vi "CAN总线测试.vi"() -> ()   [LabVIEW 2010]
panel:
  in  "同步_2":i32
  in  "同步_1":i32
  out "CAN_R_4_4":u16
  out "CAN_R_4_3":u16
  out "CAN_R_4_2":u16
  out "CAN_R_4_1":u16
  out "CAN_R_3_4":u16
  out "CAN_R_3_3":u16
  out "CAN_R_3_2":u16
  out "CAN_R_3_1":u16
  out "CAN_R_2_4":u16
  out "CAN_R_2_3":u16
  out "CAN_R_2_2":u16
  out "CAN_R_2_1":u16
  out "CAN_R_1_4":u16
  out "CAN_R_1_3":u16
  out "CAN_R_1_2":u16
  out "CAN_R_1_1":u16
  out "结束?":bool
  out "light_4":bool
  out "light_3":bool
  out "light_2":bool
  out "light_1":bool
  out "测试结论":string
  in  "btn_关闭":bool
  in  "btn_开始测试":bool
  in  "CAN_4_4":u16
  in  "CAN_4_3":u16
  in  "CAN_4_2":u16
  in  "CAN_4_1":u16
  in  "单选_CAN_4":bool
  in  "CAN_3_4":u16
  in  "CAN_3_3":u16
  in  "CAN_3_2":u16
  in  "CAN_3_1":u16
  in  "单选_CAN_3":bool
  in  "CAN_2_4":u16
  in  "CAN_2_3":u16
  in  "CAN_2_2":u16
  in  "CAN_2_1":u16
  in  "单选_CAN_2":bool
  in  "CAN_1_4":u16
  in  "CAN_1_3":u16
  in  "CAN_1_2":u16
  in  "CAN_1_1":u16
  in  "单选_CAN_1":bool
  # "CAN以发送数据："
  # "CAN1"
  # "CAN2"
  # "CAN3"
  # "CAN4"
  # "CAN接收数据："
  # "CAN1"
  # "CAN2"
  # "CAN3"
  # "CAN4"
  # "测试结论："
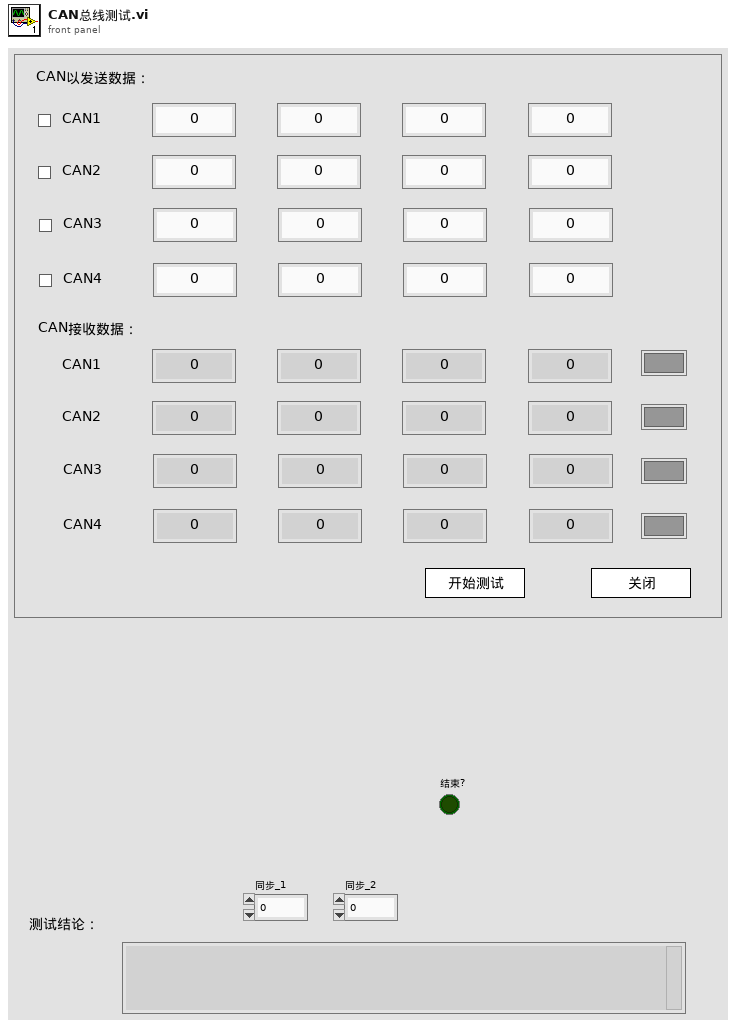
[diagram p1: front panel]
types:
  T1 = enum8{"Enabled", "Disabled", "Disabled and Grayed Out"}
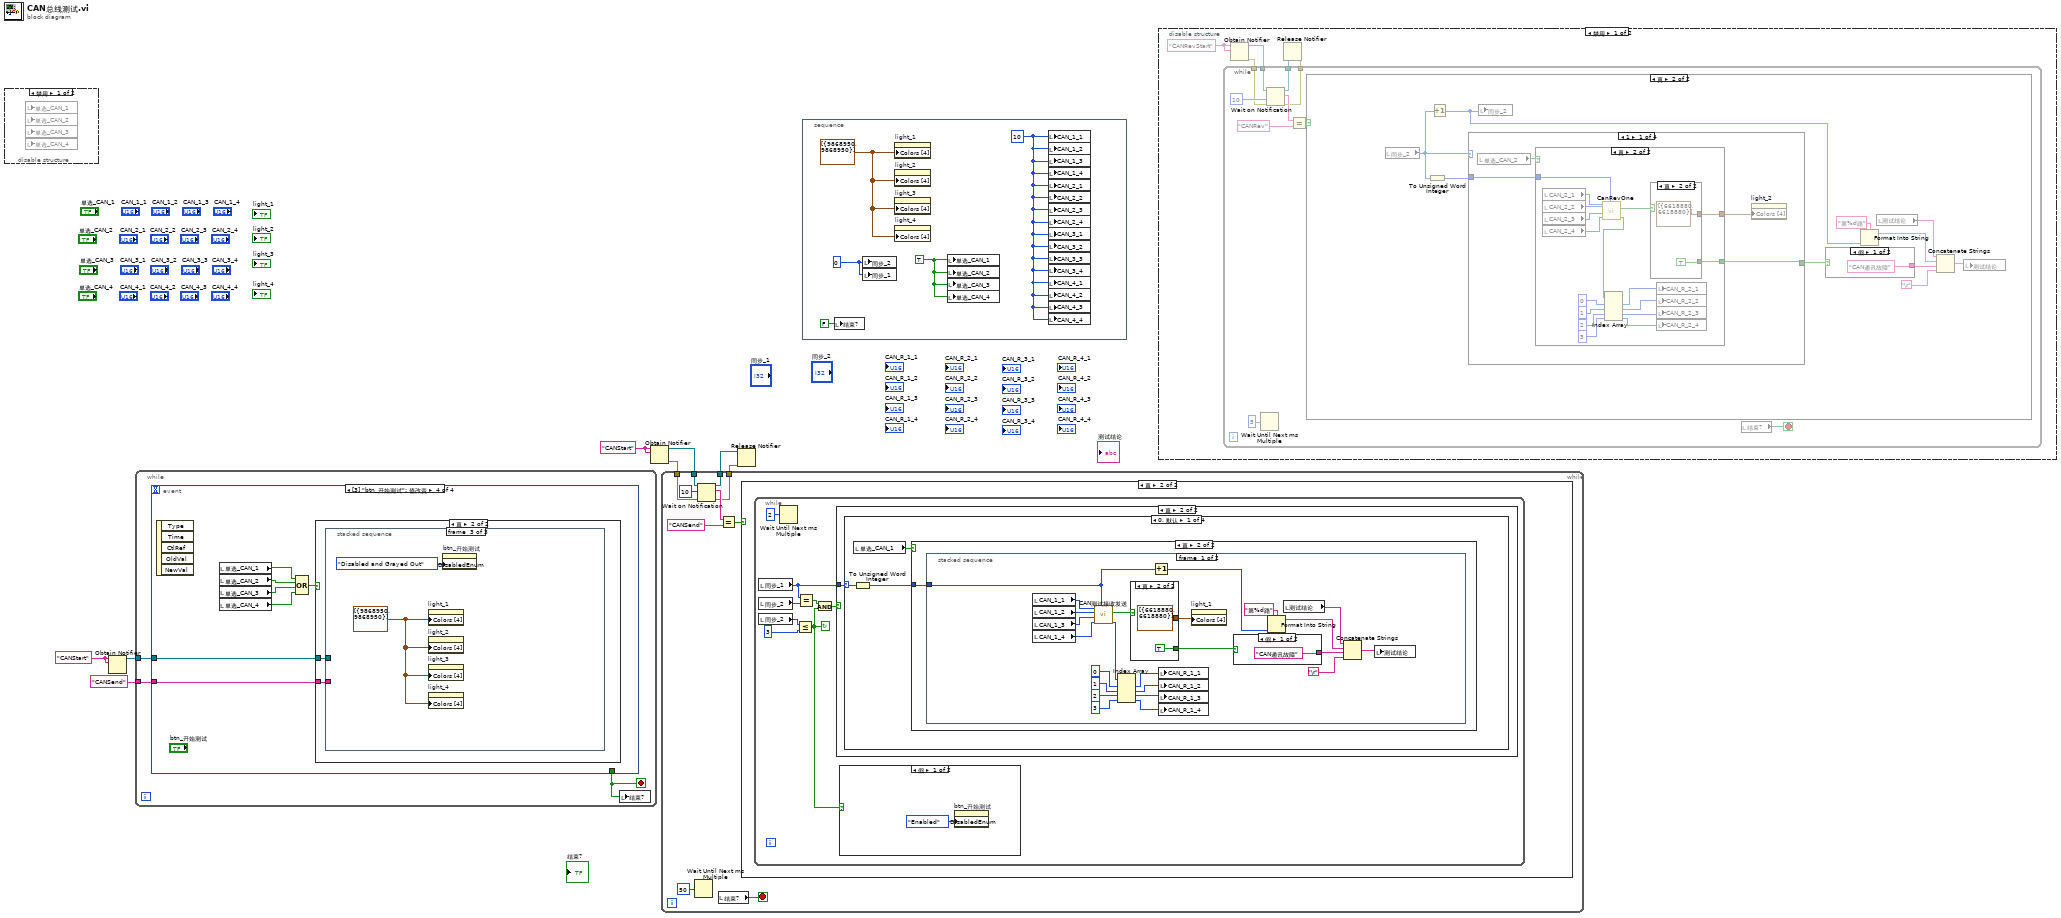
[diagram p0: block diagram]
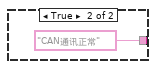
[diagram p3: hidden frame]
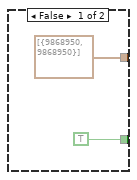
[diagram p4: hidden frame]
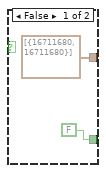
[diagram p5: hidden frame]
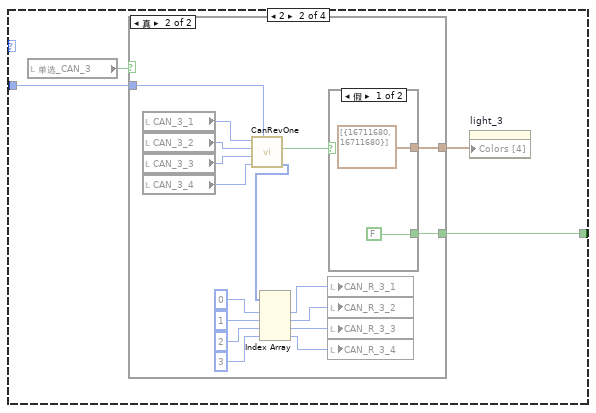
[diagram p6: hidden frame]
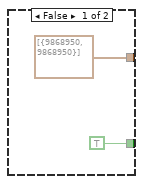
[diagram p7: hidden frame]
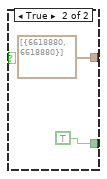
[diagram p8: hidden frame]
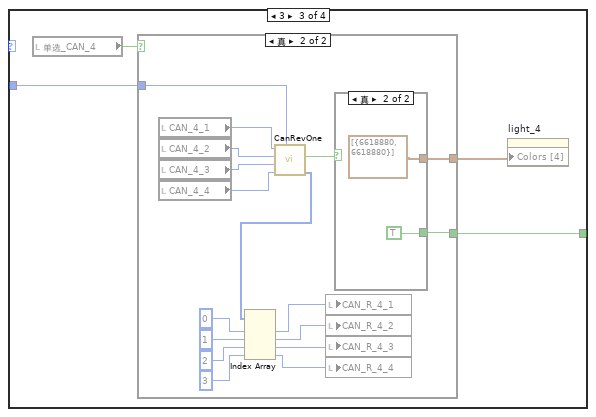
[diagram p9: hidden frame]
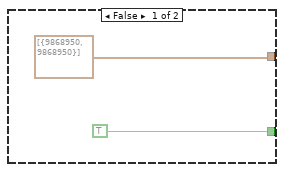
[diagram p10: hidden frame]
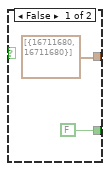
[diagram p11: hidden frame]
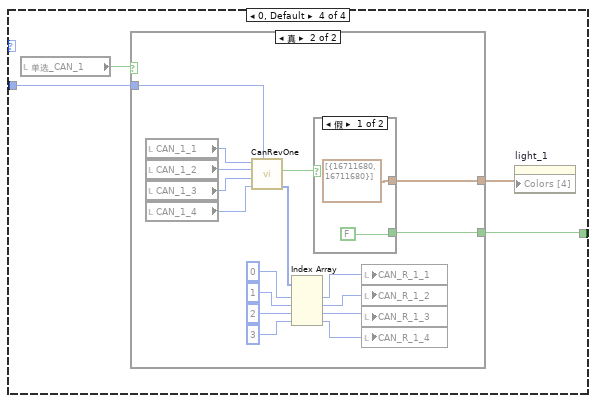
[diagram p12: hidden frame]
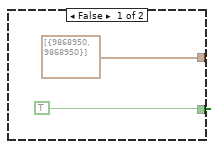
[diagram p13: hidden frame]
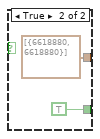
[diagram p14: hidden frame]
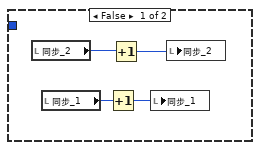
[diagram p19: hidden frame]
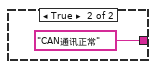
[diagram p20: hidden frame]
diagram:
  w3 = "CANStart" ("名称（未命名）")
  w8 = "CANStart" ("名称（未命名）")
  n1 = disable-structure shown="禁用" {
    frame Disabled {
      n2 = local read "单选_CAN_1"() -> ()  [unwired: 1 in]
      n3 = local read "单选_CAN_2"() -> ()  [unwired: 1 in]
      n4 = local read "单选_CAN_3"() -> ()  [unwired: 1 in]
      n5 = local read "单选_CAN_4"() -> ()  [unwired: 1 in]
    }
    frame Enabled {
    }
  }
  n6 = Obtain Notifier(name (unnamed)=w3, notification data type=w3) -> (notifier out=w2:refnum<notifier>)  [unwired: 2 in, 2 out]
  n7 = while {
    tunnel: w2 -> [w10]
    tunnel: "CANSend" ("通知") -> [w9]
    stop <- w11 stop-if-true
    n8 = event shown="[3] \"btn_开始测试\": 值改变" {
      selector: _ -> [_ _ _ _]
      dyn-events: _ -> [_ _ _ _]
      timeout: _ -> [_ _ _ _]
      tunnel: [_ TRUE TRUE _] -> w11
      tunnel: w10 -> [_ _ _ w21]
      tunnel: w9 -> [_ _ _ w20]
      event Timeout {
        n9 = event-data() -> ()  [unwired: 1 in, 2 out]
      }
      event Panel Close {
        n10 = event-data() -> ()  [unwired: 1 in, 3 out]
        n11 = stacked-sequence {
          frame #0 {
            w13 = u16 0 ("CAN_R_1_1")
            w14 = 0 ("同步_2")
            w15 = cluster{u32, u32}[] [{9868950, 9868950}]
            n12 = local write "同步_2"(w14) -> ()
            n13 = local write "同步_1"(w14) -> ()
            n14 = property on="light_1" class="Bool (严格)"("Colors [4]"=w15) -> ()  [unwired: 2 in, 2 out]
            n15 = property on="light_2" class="Bool (严格)"("Colors [4]"=w15) -> ()  [unwired: 2 in, 2 out]
            n16 = property on="light_3" class="Bool (严格)"("Colors [4]"=w15) -> ()  [unwired: 2 in, 2 out]
            n17 = property on="light_4" class="Bool (严格)"("Colors [4]"=w15) -> ()  [unwired: 2 in, 2 out]
            n18 = local write "CAN_R_1_1"(w13) -> ()
            n19 = local write "CAN_R_1_2"(w13) -> ()
            n20 = local write "CAN_R_1_3"(w13) -> ()
            n21 = local write "CAN_R_1_4"(w13) -> ()
            n22 = local write "CAN_R_2_1"(w13) -> ()
            n23 = local write "CAN_R_2_2"(w13) -> ()
            n24 = local write "CAN_R_2_3"(w13) -> ()
            n25 = local write "CAN_R_2_4"(w13) -> ()
            n26 = local write "CAN_R_3_1"(w13) -> ()
            n27 = local write "CAN_R_3_2"(w13) -> ()
            n28 = local write "CAN_R_3_3"(w13) -> ()
            n29 = local write "CAN_R_3_4"(w13) -> ()
            n30 = local write "CAN_R_4_1"(w13) -> ()
            n31 = local write "CAN_R_4_2"(w13) -> ()
            n32 = local write "CAN_R_4_3"(w13) -> ()
            n33 = local write "CAN_R_4_4"(w13) -> ()
          }
        }
      }
      event "btn_关闭": Value Change {
        n34 = event-data() -> ()  [unwired: 1 in, 5 out]
        n35 = stacked-sequence {
          frame #0 {
            w17 = u16 0 ("CAN_R_1_1")
            w18 = 0 ("同步_2")
            w19 = cluster{u32, u32}[] [{9868950, 9868950}]
            n36 = local write "同步_2"(w18) -> ()
            n37 = local write "同步_1"(w18) -> ()
            n38 = property on="light_1" class="Bool (严格)"("Colors [4]"=w19) -> ()  [unwired: 2 in, 2 out]
            n39 = property on="light_2" class="Bool (严格)"("Colors [4]"=w19) -> ()  [unwired: 2 in, 2 out]
            n40 = property on="light_3" class="Bool (严格)"("Colors [4]"=w19) -> ()  [unwired: 2 in, 2 out]
            n41 = property on="light_4" class="Bool (严格)"("Colors [4]"=w19) -> ()  [unwired: 2 in, 2 out]
            n42 = local write "CAN_R_1_1"(w17) -> ()
            n43 = local write "CAN_R_1_2"(w17) -> ()
            n44 = local write "CAN_R_1_3"(w17) -> ()
            n45 = local write "CAN_R_1_4"(w17) -> ()
            n46 = local write "CAN_R_2_1"(w17) -> ()
            n47 = local write "CAN_R_2_2"(w17) -> ()
            n48 = local write "CAN_R_2_3"(w17) -> ()
            n49 = local write "CAN_R_2_4"(w17) -> ()
            n50 = local write "CAN_R_3_1"(w17) -> ()
            n51 = local write "CAN_R_3_2"(w17) -> ()
            n52 = local write "CAN_R_3_3"(w17) -> ()
            n53 = local write "CAN_R_3_4"(w17) -> ()
            n54 = local write "CAN_R_4_1"(w17) -> ()
            n55 = local write "CAN_R_4_2"(w17) -> ()
            n56 = local write "CAN_R_4_3"(w17) -> ()
            n57 = local write "CAN_R_4_4"(w17) -> ()
          }
        }
      }
      event "btn_开始测试": Value Change {
        n58 = event-data() -> ()  [unwired: 1 in, 5 out]
        n59 = local read "单选_CAN_1"() -> (w26:bool)
        n60 = local read "单选_CAN_2"() -> (w25:bool)
        n61 = local read "单选_CAN_3"() -> (w24:bool)
        n62 = local read "单选_CAN_4"() -> (w23:bool)
        n63 = Compound Arithmetic op=OR(w26, w25, w24, w23) -> (w22:bool)
        n64 = case shown="真" w22 {
          tunnel: w21 -> [_ w28]
          tunnel: w20 -> [_ w27]
          frame False {
            n65 = call "显示对话框信息"() -> ()  [unwired: 10 in, 2 out]
          }
          frame True {
            n66 = stacked-sequence {
              tunnel: w28 -> [_ w33 _]
              tunnel: w27 -> [_ w32 _]
              frame #0 {
                w29 = u16 0 ("CAN_R_1_1")
                w30 = 0 ("同步_2")
                n67 = local write "同步_2"(w30) -> ()
                n68 = local write "同步_1"(w30) -> ()
                n69 = local write "测试结论"("") -> ()
                n70 = local write "CAN_R_1_1"(w29) -> ()
                n71 = local write "CAN_R_1_2"(w29) -> ()
                n72 = local write "CAN_R_1_3"(w29) -> ()
                n73 = local write "CAN_R_1_4"(w29) -> ()
                n74 = local write "CAN_R_2_1"(w29) -> ()
                n75 = local write "CAN_R_2_2"(w29) -> ()
                n76 = local write "CAN_R_2_3"(w29) -> ()
                n77 = local write "CAN_R_2_4"(w29) -> ()
                n78 = local write "CAN_R_3_1"(w29) -> ()
                n79 = local write "CAN_R_3_2"(w29) -> ()
                n80 = local write "CAN_R_3_3"(w29) -> ()
                n81 = local write "CAN_R_3_4"(w29) -> ()
                n82 = local write "CAN_R_4_1"(w29) -> ()
                n83 = local write "CAN_R_4_2"(w29) -> ()
                n84 = local write "CAN_R_4_3"(w29) -> ()
                n85 = local write "CAN_R_4_4"(w29) -> ()
              }
              frame #1 {
                n86 = Send Notification(notification=w32, notifier=w33) -> ()  [unwired: 1 in, 2 out]
              }
              frame #2 {
                w34 = cluster{u32, u32}[] [{9868950, 9868950}]
                n87 = property on="light_1" class="Bool (严格)"("Colors [4]"=w34) -> ()  [unwired: 2 in, 2 out]
                n88 = property on="light_2" class="Bool (严格)"("Colors [4]"=w34) -> ()  [unwired: 2 in, 2 out]
                n89 = property on="light_3" class="Bool (严格)"("Colors [4]"=w34) -> ()  [unwired: 2 in, 2 out]
                n90 = property on="light_4" class="Bool (严格)"("Colors [4]"=w34) -> ()  [unwired: 2 in, 2 out]
                n91 = property on="btn_开始测试" class="Bool"("DisabledEnum"=T1."Disabled and Grayed Out" ("禁用")) -> ()  [unwired: 2 in, 2 out]
              }
            }
          }
        }
      }
    }
    n92 = local write "结束?"(w11) -> ()
  }
  n93 = Obtain Notifier(name (unnamed)=w8, notification data type=w8) -> (notifier out=w6:refnum<notifier>, error out=w7:errorcluster)  [unwired: 2 in, 1 out]
  n94 = while {
    tunnel: w7 -> [w39]
    tunnel: w6 -> [w38]
    tunnel: [w37] -> w5
    tunnel: [w36] -> w4
    stop <- w44 stop-if-true
    n95 = Wait Until Next ms Multiple(millisecond multiple=u32 50 ("毫秒倍数")) -> ()  [unwired: 1 out]
    n96 = Wait on Notification(notifier=w38, timeout in ms (-1)=10 ("超时毫秒(-1)"), error in (no error)=w39) -> (notifier out=w37:refnum<notifier>, notification=w41:string, error out=w36:errorcluster)  [unwired: 1 in, 1 out]
    n97 = local read "结束?"() -> (w44:bool)
    n98 = Equal?(x=w41, y="CANSend" ("通知")) -> (x = y?=w40:bool)
    n99 = case shown="真" w40 {
      frame False {
      }
      frame True {
        n100 = while {
          stop <- w46 continue-if-true
          n101 = local read "同步_1"() -> (w53:i32)
          n102 = local read "同步_2"() -> (w49:i32)
          n103 = local read "同步_2"() -> (w51:i32)
          n104 = Wait Until Next ms Multiple(millisecond multiple=u32 2 ("毫秒倍数")) -> ()  [unwired: 1 out]
          n105 = Less Or Equal?(x=w51, y=3) -> (x <= y?=w46:bool)
          n106 = Equal?(x=w53, y=w49) -> (x = y?=w47:bool)
          n107 = And(x=w47, y=w46) -> (x .and. y?=w48:bool)
          n108 = case shown="真" w48 {
            tunnel: w53 -> [_ w55]
            frame False {
            }
            frame True {
              n109 = case shown="0, 默认" w55 {
                selector: w55 -> [w56 w100 w142 w184]
                frame 0, Default {
                  n110 = local read "单选_CAN_1"() -> (w58:bool)
                  n111 = To Unsigned Word Integer(number=w56) -> (unsigned 16bit integer=w57:u16)
                  n112 = case shown="真" w58 {
                    tunnel: w57 -> [_ w63]
                    frame False {
                      n113 = local read "同步_2"() -> (w61:i32)
                      n114 = local read "同步_1"() -> (w59:i32)
                      n115 = Increment(x=w59) -> (x+1=w60:i32)
                      n116 = Increment(x=w61) -> (x+1=w62:i32)
                      n117 = local write "同步_1"(w60) -> ()
                      n118 = local write "同步_2"(w62) -> ()
                    }
                    frame True {
                      n119 = stacked-sequence {
                        tunnel: w63 -> [w64 _]
                        frame #0 {
                          n120 = local read "CAN_1_1"() -> (w74:u16)
                          n121 = local read "CAN_1_2"() -> (w75:u16)
                          n122 = local read "CAN_1_3"() -> (w76:u16)
                          n123 = local read "CAN_1_4"() -> (w77:u16)
                          n124 = call "CAN测试接收发送.vi"("Order"=w64, "data_4"=w77, "data_3"=w76, "data_2"=w75, "data_1"=w74) -> ("接收数据"=w79:u16[], "成功？"=w78:bool)  [unwired: 5 in]
                          n125 = Index Array(array=w79, index #1=0 ("索引"), index #2=1 ("索引"), index #3=2 ("索引"), index #4=3 ("索引")) -> (element #1=w84:u16, element #2=w85:u16, element #3=w86:u16, element #4=w87:u16)
                          n126 = case shown="真" w78 {
                            tunnel: [cluster{u32, u32}[] [{16711680, 16711680}] cluster{u32, u32}[] [{6618880, 6618880}]] -> w73
                            tunnel: [FALSE TRUE] -> w65
                            frame False {
                            }
                            frame True {
                            }
                          }
                          n127 = Increment(x=w64) -> (x+1=w66:u16)
                          n128 = local write "CAN_R_1_1"(w84) -> ()
                          n129 = local write "CAN_R_1_2"(w85) -> ()
                          n130 = local write "CAN_R_1_3"(w86) -> ()
                          n131 = local write "CAN_R_1_4"(w87) -> ()
                          n132 = property on="light_1" class="Bool (严格)"("Colors [4]"=w73) -> ()  [unwired: 2 in, 2 out]
                          n133 = case shown="假" w65 {
                            tunnel: ["CAN通讯故障" "CAN通讯正常"] -> w69
                            frame False {
                            }
                            frame True {
                            }
                          }
                          n134 = Format Into String(format string="第%d路", w66) -> (resulting string=w70:string)  [unwired: 2 in, 1 out]
                          n135 = local read "测试结论"() -> (w71:string)
                          n136 = Concatenate Strings(w71, w70, w69, "\r") -> (w67:string)
                          n137 = local write "测试结论"(w67) -> ()
                        }
                        frame #1 {
                          n138 = local read "同步_1"() -> (w96:i32)
                          n139 = local read "同步_2"() -> (w94:i32)
                          n140 = Increment(x=w96) -> (x+1=w97:i32)
                          n141 = Increment(x=w94) -> (x+1=w95:i32)
                          n142 = local write "同步_2"(w95) -> ()
                          n143 = local write "同步_1"(w97) -> ()
                        }
                      }
                    }
                  }
                }
                frame 1 {
                  n144 = local read "单选_CAN_2"() -> (w99:bool)
                  n145 = To Unsigned Word Integer(number=w100) -> (unsigned 16bit integer=w98:u16)
                  n146 = case shown="真" w99 {
                    tunnel: w98 -> [_ w105]
                    frame False {
                      n147 = local read "同步_2"() -> (w103:i32)
                      n148 = local read "同步_1"() -> (w101:i32)
                      n149 = Increment(x=w101) -> (x+1=w102:i32)
                      n150 = Increment(x=w103) -> (x+1=w104:i32)
                      n151 = local write "同步_1"(w102) -> ()
                      n152 = local write "同步_2"(w104) -> ()
                    }
                    frame True {
                      n153 = stacked-sequence {
                        tunnel: w105 -> [w129 _]
                        frame #0 {
                          n154 = local read "CAN_2_1"() -> (w115:u16)
                          n155 = local read "CAN_2_2"() -> (w116:u16)
                          n156 = local read "CAN_2_3"() -> (w117:u16)
                          n157 = local read "CAN_2_4"() -> (w118:u16)
                          n158 = call "CAN测试接收发送.vi"("Order"=w129, "data_4"=w118, "data_3"=w117, "data_2"=w116, "data_1"=w115) -> ("接收数据"=w124:u16[], "成功？"=w119:bool)  [unwired: 5 in]
                          n159 = Index Array(array=w124, index #1=0 ("索引"), index #2=1 ("索引"), index #3=2 ("索引"), index #4=3 ("索引")) -> (element #1=w125:u16, element #2=w126:u16, element #3=w127:u16, element #4=w128:u16)
                          n160 = case shown="真" w119 {
                            tunnel: [cluster{u32, u32}[] [{16711680, 16711680}] cluster{u32, u32}[] [{6618880, 6618880}]] -> w114
                            tunnel: [FALSE TRUE] -> w107
                            frame False {
                            }
                            frame True {
                            }
                          }
                          n161 = local write "CAN_R_2_1"(w125) -> ()
                          n162 = local write "CAN_R_2_2"(w126) -> ()
                          n163 = local write "CAN_R_2_3"(w127) -> ()
                          n164 = local write "CAN_R_2_4"(w128) -> ()
                          n165 = Increment(x=w129) -> (x+1=w106:u16)
                          n166 = property on="light_2" class="Bool (严格)"("Colors [4]"=w114) -> ()  [unwired: 2 in, 2 out]
                          n167 = case shown="假" w107 {
                            tunnel: ["CAN通讯故障" "CAN通讯正常"] -> w111
                            frame False {
                            }
                            frame True {
                            }
                          }
                          n168 = Format Into String(format string="第%d路", w106) -> (resulting string=w110:string)  [unwired: 2 in, 1 out]
                          n169 = local read "测试结论"() -> (w109:string)
                          n170 = Concatenate Strings(w109, w110, w111, "\r") -> (w113:string)
                          n171 = local write "测试结论"(w113) -> ()
                        }
                        frame #1 {
                          n172 = local read "同步_1"() -> (w138:i32)
                          n173 = local read "同步_2"() -> (w137:i32)
                          n174 = Increment(x=w138) -> (x+1=w139:i32)
                          n175 = Increment(x=w137) -> (x+1=w136:i32)
                          n176 = local write "同步_2"(w136) -> ()
                          n177 = local write "同步_1"(w139) -> ()
                        }
                      }
                    }
                  }
                }
                frame 2 {
                  n178 = local read "单选_CAN_3"() -> (w141:bool)
                  n179 = To Unsigned Word Integer(number=w142) -> (unsigned 16bit integer=w140:u16)
                  n180 = case shown="真" w141 {
                    tunnel: w140 -> [_ w147]
                    frame False {
                      n181 = local read "同步_1"() -> (w143:i32)
                      n182 = local read "同步_2"() -> (w145:i32)
                      n183 = Increment(x=w143) -> (x+1=w144:i32)
                      n184 = Increment(x=w145) -> (x+1=w146:i32)
                      n185 = local write "同步_1"(w144) -> ()
                      n186 = local write "同步_2"(w146) -> ()
                    }
                    frame True {
                      n187 = stacked-sequence {
                        tunnel: w147 -> [w171 _]
                        frame #0 {
                          n188 = local read "CAN_3_1"() -> (w157:u16)
                          n189 = local read "CAN_3_2"() -> (w158:u16)
                          n190 = local read "CAN_3_3"() -> (w159:u16)
                          n191 = local read "CAN_3_4"() -> (w160:u16)
                          n192 = call "CAN测试接收发送.vi"("Order"=w171, "data_4"=w160, "data_3"=w159, "data_2"=w158, "data_1"=w157) -> ("接收数据"=w166:u16[], "成功？"=w161:bool)  [unwired: 5 in]
                          n193 = Index Array(array=w166, index #1=0 ("索引"), index #2=1 ("索引"), index #3=2 ("索引"), index #4=3 ("索引")) -> (element #1=w167:u16, element #2=w168:u16, element #3=w169:u16, element #4=w170:u16)
                          n194 = local write "CAN_R_3_1"(w167) -> ()
                          n195 = local write "CAN_R_3_2"(w168) -> ()
                          n196 = local write "CAN_R_3_3"(w169) -> ()
                          n197 = local write "CAN_R_3_4"(w170) -> ()
                          n198 = case shown="真" w161 {
                            tunnel: [cluster{u32, u32}[] [{16711680, 16711680}] cluster{u32, u32}[] [{6618880, 6618880}]] -> w156
                            tunnel: [FALSE TRUE] -> w148
                            frame False {
                            }
                            frame True {
                            }
                          }
                          n199 = Increment(x=w171) -> (x+1=w149:u16)
                          n200 = property on="light_3" class="Bool (严格)"("Colors [4]"=w156) -> ()  [unwired: 2 in, 2 out]
                          n201 = case shown="假" w148 {
                            tunnel: ["CAN通讯故障" "CAN通讯正常"] -> w153
                            frame False {
                            }
                            frame True {
                            }
                          }
                          n202 = Format Into String(format string="第%d路", w149) -> (resulting string=w152:string)  [unwired: 2 in, 1 out]
                          n203 = local read "测试结论"() -> (w151:string)
                          n204 = Concatenate Strings(w151, w152, w153, "\r") -> (w155:string)
                          n205 = local write "测试结论"(w155) -> ()
                        }
                        frame #1 {
                          n206 = local read "同步_1"() -> (w180:i32)
                          n207 = local read "同步_2"() -> (w178:i32)
                          n208 = Increment(x=w180) -> (x+1=w181:i32)
                          n209 = Increment(x=w178) -> (x+1=w179:i32)
                          n210 = local write "同步_1"(w181) -> ()
                          n211 = local write "同步_2"(w179) -> ()
                        }
                      }
                    }
                  }
                }
                frame 3 {
                  n212 = local read "单选_CAN_4"() -> (w183:bool)
                  n213 = To Unsigned Word Integer(number=w184) -> (unsigned 16bit integer=w182:u16)
                  n214 = case shown="真" w183 {
                    tunnel: w182 -> [_ w189]
                    frame False {
                      n215 = local read "同步_2"() -> (w187:i32)
                      n216 = local read "同步_1"() -> (w186:i32)
                      n217 = Increment(x=w187) -> (x+1=w188:i32)
                      n218 = Increment(x=w186) -> (x+1=w185:i32)
                      n219 = local write "同步_1"(w185) -> ()
                      n220 = local write "同步_2"(w188) -> ()
                    }
                    frame True {
                      n221 = stacked-sequence {
                        tunnel: w189 -> [w213 _]
                        frame #0 {
                          n222 = local read "CAN_4_1"() -> (w212:u16)
                          n223 = local read "CAN_4_2"() -> (w211:u16)
                          n224 = local read "CAN_4_3"() -> (w210:u16)
                          n225 = local read "CAN_4_4"() -> (w209:u16)
                          n226 = call "CAN测试接收发送.vi"("Order"=w213, "data_4"=w209, "data_3"=w210, "data_2"=w211, "data_1"=w212) -> ("接收数据"=w203:u16[], "成功？"=w208:bool)  [unwired: 5 in]
                          n227 = Index Array(array=w203, index #1=0 ("索引"), index #2=1 ("索引"), index #3=2 ("索引"), index #4=3 ("索引")) -> (element #1=w202:u16, element #2=w201:u16, element #3=w200:u16, element #4=w199:u16)
                          n228 = local write "CAN_R_4_1"(w202) -> ()
                          n229 = local write "CAN_R_4_2"(w201) -> ()
                          n230 = local write "CAN_R_4_3"(w200) -> ()
                          n231 = local write "CAN_R_4_4"(w199) -> ()
                          n232 = case shown="真" w208 {
                            tunnel: [cluster{u32, u32}[] [{16711680, 16711680}] cluster{u32, u32}[] [{6618880, 6618880}]] -> w198
                            tunnel: [FALSE TRUE] -> w190
                            frame False {
                            }
                            frame True {
                            }
                          }
                          n233 = Increment(x=w213) -> (x+1=w191:u16)
                          n234 = property on="light_4" class="Bool (严格)"("Colors [4]"=w198) -> ()  [unwired: 2 in, 2 out]
                          n235 = case shown="假" w190 {
                            tunnel: ["CAN通讯故障" "CAN通讯正常"] -> w195
                            frame False {
                            }
                            frame True {
                            }
                          }
                          n236 = Format Into String(format string="第%d路", w191) -> (resulting string=w194:string)  [unwired: 2 in, 1 out]
                          n237 = local read "测试结论"() -> (w193:string)
                          n238 = Concatenate Strings(w193, w194, w195, "\r") -> (w197:string)
                          n239 = local write "测试结论"(w197) -> ()
                        }
                        frame #1 {
                          n240 = local read "同步_1"() -> (w223:i32)
                          n241 = local read "同步_2"() -> (w220:i32)
                          n242 = Increment(x=w223) -> (x+1=w222:i32)
                          n243 = Increment(x=w220) -> (x+1=w221:i32)
                          n244 = local write "同步_2"(w221) -> ()
                          n245 = local write "同步_1"(w222) -> ()
                        }
                      }
                    }
                  }
                }
              }
            }
          }
          n246 = case shown="假" w46 {
            frame False {
              n247 = property on="btn_开始测试" class="Bool"("DisabledEnum"=T1."Enabled" ("禁用")) -> ()  [unwired: 2 in, 2 out]
            }
            frame True {
            }
          }
        }
      }
    }
  }
  n248 = Release Notifier(notifier=w5, error in (no error)=w4) -> ()  [unwired: 1 in, 3 out]
  n249 = stacked-sequence {
    frame #0 {
      w224 = TRUE ("单选_CAN_1")
      w225 = u16 10 ("CAN_R_1_1")
      w226 = 0 ("同步_2")
      w228 = cluster{u32, u32}[] [{9868950, 9868950}]
      n250 = local write "结束?"(FALSE ("结束?")) -> ()
      n251 = local write "同步_2"(w226) -> ()
      n252 = local write "同步_1"(w226) -> ()
      n253 = property on="light_1" class="Bool (严格)"("Colors [4]"=w228) -> ()  [unwired: 2 in, 2 out]
      n254 = property on="light_2" class="Bool (严格)"("Colors [4]"=w228) -> ()  [unwired: 2 in, 2 out]
      n255 = property on="light_3" class="Bool (严格)"("Colors [4]"=w228) -> ()  [unwired: 2 in, 2 out]
      n256 = property on="light_4" class="Bool (严格)"("Colors [4]"=w228) -> ()  [unwired: 2 in, 2 out]
      n257 = local write "单选_CAN_1"(w224) -> ()
      n258 = local write "单选_CAN_2"(w224) -> ()
      n259 = local write "单选_CAN_3"(w224) -> ()
      n260 = local write "单选_CAN_4"(w224) -> ()
      n261 = local write "CAN_1_1"(w225) -> ()
      n262 = local write "CAN_1_2"(w225) -> ()
      n263 = local write "CAN_1_3"(w225) -> ()
      n264 = local write "CAN_1_4"(w225) -> ()
      n265 = local write "CAN_2_1"(w225) -> ()
      n266 = local write "CAN_2_2"(w225) -> ()
      n267 = local write "CAN_2_3"(w225) -> ()
      n268 = local write "CAN_2_4"(w225) -> ()
      n269 = local write "CAN_3_1"(w225) -> ()
      n270 = local write "CAN_3_2"(w225) -> ()
      n271 = local write "CAN_3_3"(w225) -> ()
      n272 = local write "CAN_3_4"(w225) -> ()
      n273 = local write "CAN_4_1"(w225) -> ()
      n274 = local write "CAN_4_2"(w225) -> ()
      n275 = local write "CAN_4_3"(w225) -> ()
      n276 = local write "CAN_4_4"(w225) -> ()
    }
  }
  n277 = disable-structure shown="禁用" {
    frame Disabled {
      w233 = "CANRevStart" ("名称（未命名）")
      n278 = Obtain Notifier(name (unnamed)=w233, notification data type=w233) -> (notifier out=w231:refnum<notifier>, error out=w232:errorcluster)  [unwired: 2 in, 1 out]
      n279 = while {
        tunnel: w232 -> [w238]
        tunnel: w231 -> [w237]
        tunnel: [w236] -> w230
        tunnel: [w235] -> w229
        stop <- w243 stop-if-true
        n280 = Wait Until Next ms Multiple(millisecond multiple=u32 5 ("毫秒倍数")) -> ()  [unwired: 1 out]
        n281 = Wait on Notification(notifier=w237, timeout in ms (-1)=10 ("超时毫秒(-1)"), error in (no error)=w238) -> (notifier out=w236:refnum<notifier>, notification=w240:string, error out=w235:errorcluster)  [unwired: 1 in, 1 out]
        n282 = Equal?(x=w240, y="CANRev" ("通知")) -> (x = y?=w234:bool)
        n283 = case shown="真" w234 {
          frame False {
          }
          frame True {
            n284 = local read "同步_2"() -> (w253:i32)
            n285 = To Unsigned Word Integer(number=w253) -> (unsigned 16bit integer=w252:u16)
            n286 = Increment(x=w253) -> (x+1=w245:i32)
            n287 = case shown="1" w253 {
              tunnel: w252 -> [w258 w285 w312 w339]
              tunnel: [w256 w283 w310 w337] -> w246
              frame 1 {
                n288 = local read "单选_CAN_2"() -> (w259:bool)
                n289 = case shown="真" w259 {
                  tunnel: w258 -> [_ w278]
                  tunnel: [TRUE w272] -> w256
                  tunnel: [cluster{u32, u32}[] [{9868950, 9868950}] w266] -> w257
                  frame False {
                  }
                  frame True {
                    n290 = local read "CAN_2_1"() -> (w277:u16)
                    n291 = local read "CAN_2_2"() -> (w276:u16)
                    n292 = local read "CAN_2_3"() -> (w275:u16)
                    n293 = local read "CAN_2_4"() -> (w274:u16)
                    n294 = call "CanRevOne.vi"("CANPort"=w278, "data_4"=w274, "data_3"=w275, "data_2"=w276, "data_1"=w277) -> ("接收数据"=w267:u16[], "成功？"=w273:bool)  [unwired: 5 in]
                    n295 = Index Array(array=w267, index #1=0 ("索引"), index #2=1 ("索引"), index #3=2 ("索引"), index #4=3 ("索引")) -> (element #1=w265:u16, element #2=w264:u16, element #3=w263:u16, element #4=w262:u16)
                    n296 = case shown="真" w273 {
                      tunnel: [cluster{u32, u32}[] [{16711680, 16711680}] cluster{u32, u32}[] [{6618880, 6618880}]] -> w266
                      tunnel: [FALSE TRUE] -> w272
                      frame False {
                      }
                      frame True {
                      }
                    }
                    n297 = local write "CAN_R_2_1"(w265) -> ()
                    n298 = local write "CAN_R_2_2"(w264) -> ()
                    n299 = local write "CAN_R_2_3"(w263) -> ()
                    n300 = local write "CAN_R_2_4"(w262) -> ()
                  }
                }
                n301 = property on="light_2" class="Bool (严格)"("Colors [4]"=w257) -> ()  [unwired: 2 in, 2 out]
              }
              frame 2 {
                n302 = local read "单选_CAN_3"() -> (w286:bool)
                n303 = case shown="真" w286 {
                  tunnel: w285 -> [_ w305]
                  tunnel: [TRUE w299] -> w283
                  tunnel: [cluster{u32, u32}[] [{9868950, 9868950}] w293] -> w284
                  frame False {
                  }
                  frame True {
                    n304 = local read "CAN_3_1"() -> (w304:u16)
                    n305 = local read "CAN_3_2"() -> (w303:u16)
                    n306 = local read "CAN_3_3"() -> (w302:u16)
                    n307 = local read "CAN_3_4"() -> (w301:u16)
                    n308 = call "CanRevOne.vi"("CANPort"=w305, "data_4"=w301, "data_3"=w302, "data_2"=w303, "data_1"=w304) -> ("接收数据"=w294:u16[], "成功？"=w300:bool)  [unwired: 5 in]
                    n309 = Index Array(array=w294, index #1=0 ("索引"), index #2=1 ("索引"), index #3=2 ("索引"), index #4=3 ("索引")) -> (element #1=w292:u16, element #2=w291:u16, element #3=w290:u16, element #4=w289:u16)
                    n310 = local write "CAN_R_3_1"(w292) -> ()
                    n311 = local write "CAN_R_3_2"(w291) -> ()
                    n312 = local write "CAN_R_3_3"(w290) -> ()
                    n313 = local write "CAN_R_3_4"(w289) -> ()
                    n314 = case shown="假" w300 {
                      tunnel: [cluster{u32, u32}[] [{16711680, 16711680}] cluster{u32, u32}[] [{6618880, 6618880}]] -> w293
                      tunnel: [FALSE TRUE] -> w299
                      frame False {
                      }
                      frame True {
                      }
                    }
                  }
                }
                n315 = property on="light_3" class="Bool (严格)"("Colors [4]"=w284) -> ()  [unwired: 2 in, 2 out]
              }
              frame 3 {
                n316 = local read "单选_CAN_4"() -> (w313:bool)
                n317 = case shown="真" w313 {
                  tunnel: w312 -> [_ w332]
                  tunnel: [TRUE w326] -> w310
                  tunnel: [cluster{u32, u32}[] [{9868950, 9868950}] w320] -> w311
                  frame False {
                  }
                  frame True {
                    n318 = local read "CAN_4_1"() -> (w331:u16)
                    n319 = local read "CAN_4_2"() -> (w330:u16)
                    n320 = local read "CAN_4_3"() -> (w329:u16)
                    n321 = local read "CAN_4_4"() -> (w328:u16)
                    n322 = call "CanRevOne.vi"("CANPort"=w332, "data_4"=w328, "data_3"=w329, "data_2"=w330, "data_1"=w331) -> ("接收数据"=w321:u16[], "成功？"=w327:bool)  [unwired: 5 in]
                    n323 = Index Array(array=w321, index #1=0 ("索引"), index #2=1 ("索引"), index #3=2 ("索引"), index #4=3 ("索引")) -> (element #1=w319:u16, element #2=w318:u16, element #3=w317:u16, element #4=w316:u16)
                    n324 = local write "CAN_R_4_1"(w319) -> ()
                    n325 = local write "CAN_R_4_2"(w318) -> ()
                    n326 = local write "CAN_R_4_3"(w317) -> ()
                    n327 = local write "CAN_R_4_4"(w316) -> ()
                    n328 = case shown="真" w327 {
                      tunnel: [cluster{u32, u32}[] [{16711680, 16711680}] cluster{u32, u32}[] [{6618880, 6618880}]] -> w320
                      tunnel: [FALSE TRUE] -> w326
                      frame False {
                      }
                      frame True {
                      }
                    }
                  }
                }
                n329 = property on="light_4" class="Bool (严格)"("Colors [4]"=w311) -> ()  [unwired: 2 in, 2 out]
              }
              frame 0, Default {
                n330 = local read "单选_CAN_1"() -> (w340:bool)
                n331 = case shown="真" w340 {
                  tunnel: w339 -> [_ w359]
                  tunnel: [TRUE w353] -> w337
                  tunnel: [cluster{u32, u32}[] [{9868950, 9868950}] w347] -> w338
                  frame False {
                  }
                  frame True {
                    n332 = local read "CAN_1_1"() -> (w358:u16)
                    n333 = local read "CAN_1_2"() -> (w357:u16)
                    n334 = local read "CAN_1_3"() -> (w356:u16)
                    n335 = local read "CAN_1_4"() -> (w355:u16)
                    n336 = call "CanRevOne.vi"("CANPort"=w359, "data_4"=w355, "data_3"=w356, "data_2"=w357, "data_1"=w358) -> ("接收数据"=w352:u16[], "成功？"=w354:bool)  [unwired: 5 in]
                    n337 = Index Array(array=w352, index #1=0 ("索引"), index #2=1 ("索引"), index #3=2 ("索引"), index #4=3 ("索引")) -> (element #1=w346:u16, element #2=w345:u16, element #3=w344:u16, element #4=w343:u16)
                    n338 = case shown="假" w354 {
                      tunnel: [cluster{u32, u32}[] [{16711680, 16711680}] cluster{u32, u32}[] [{6618880, 6618880}]] -> w347
                      tunnel: [FALSE TRUE] -> w353
                      frame False {
                      }
                      frame True {
                      }
                    }
                    n339 = local write "CAN_R_1_1"(w346) -> ()
                    n340 = local write "CAN_R_1_2"(w345) -> ()
                    n341 = local write "CAN_R_1_3"(w344) -> ()
                    n342 = local write "CAN_R_1_4"(w343) -> ()
                  }
                }
                n343 = property on="light_1" class="Bool (严格)"("Colors [4]"=w338) -> ()  [unwired: 2 in, 2 out]
              }
            }
            n344 = local write "同步_2"(w245) -> ()
            n345 = case shown="假" w246 {
              tunnel: ["CAN通讯故障" "CAN通讯正常"] -> w248
              frame False {
              }
              frame True {
              }
            }
            n346 = Format Into String(format string="第%d路", w245) -> (resulting string=w249:string)  [unwired: 2 in, 1 out]
            n347 = local read "测试结论"() -> (w250:string)
            n348 = Concatenate Strings(w250, w249, w248, "\r") -> (w244:string)
            n349 = local write "测试结论"(w244) -> ()
          }
        }
        n350 = local read "结束?"() -> (w243:bool)
      }
      n351 = Release Notifier(notifier=w230, error in (no error)=w229) -> ()  [unwired: 1 in, 3 out]
    }
    frame Enabled {
    }
  }
